vi "TDC_getTimestampBufferSize.vi"(8 "Error In":errorcluster) -> (0 "Error Out":errorcluster, 3 "Buffer Size":i32)   [LabVIEW 2011]
uses:
  tdcbase.dll
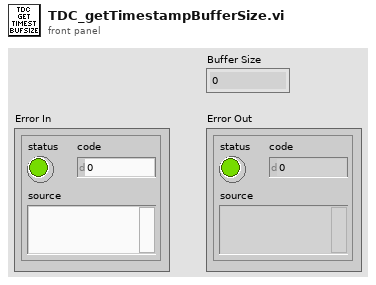
[diagram p1: front panel]
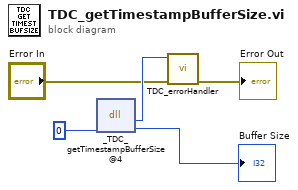
[diagram p0: block diagram]
diagram:
  n1 = dll-call lib="X:/tdcbase.dll" fn="_TDC_getTimestampBufferSize@4"("size"=0) -> ("return type"=w3:i32, "size"=→"Buffer Size":i32)  [unwired: 3 in, 2 out]
  n2 = call "TDC_errorHandler.vi"("Error In"="Error In", "TDC Return Code"=w3) -> ("Error Out"=→"Error Out":errorcluster)  [unwired: 9 in]
